vi "Lecture5exercise1.vi"() -> ()   [LabVIEW 2022 SP3]
uses:
  <vilib>/sound2/lvsound2.llb/Sampling Mode.ctl
  <vilib>/Analysis/2dsp.llb/Real FFT.vi
  <vilib>/sound2/lvsound2.llb/Sound Input Read (DBL).vi
  <vilib>/Analysis/NI_AALPro.lvlib
panel:
  out "Numeric":dbl
  out "Frequency Spectrum":cluster{dbl, dbl, dbl[]}(graph)
  out "Waveform Graph":waveform(dbl)(graph)
  in  "stop":bool
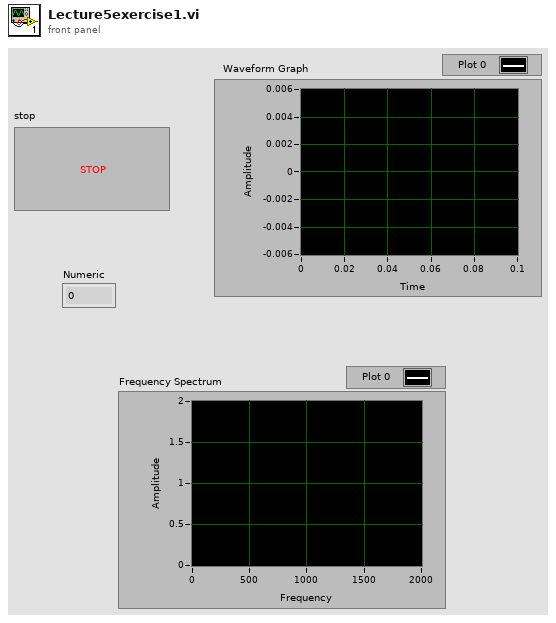
[diagram p1: front panel]
types:
  T1 = typedef "Sampling Mode.ctl" = i32
  T2 = typedef "Sound Input Task ID.ctl" = u32
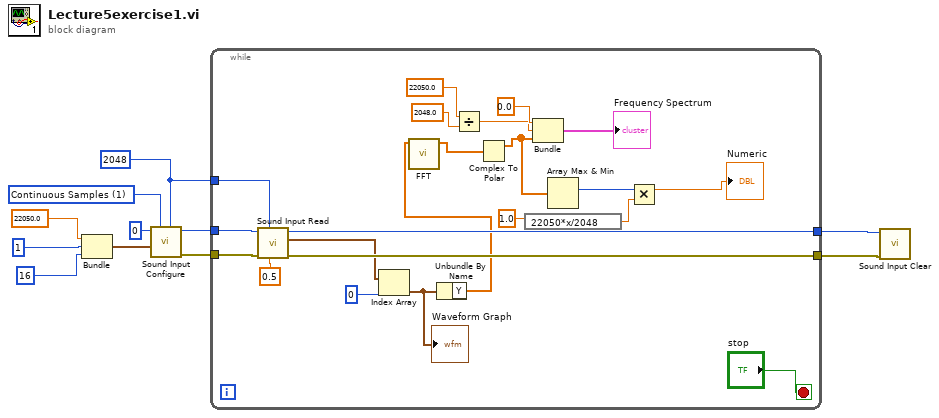
[diagram p0: block diagram]
diagram:
  w3 = 2048 ("number of samples/ch")
  w6 = T1 1 items=["Finite Samples", "Continuous Samples"] ("sample mode")
  n1 = Bundle(22050.0, 1, 16) -> (w8:cluster{dbl, i32, i32})  [unwired: 1 in]
  n2 = call <vilib>:"Sound Input Configure.vi"("number of samples/ch"=w3, "sample mode"=w6, "sound format"=w8, "device ID"=u32 0) -> ("error out"=w5:errorcluster, "task ID"=w4:T2)  [unwired: 6 in]
  n3 = while {
    tunnel: w5 -> [w29]
    tunnel: w4 -> [w28]
    tunnel: w3 -> [w27]
    tunnel: [w26] -> w2
    tunnel: [w25] -> w1
    stop <- "stop" stop-if-true
    n4 = call-poly <vilib>:"Sound Input Read.vi"("timeout (sec)"=0.5, "number of samples/ch"=w27, "error in (no error)"=w29, "task ID"=w28) -> ("error out"=w25:errorcluster, "data"=w24:waveform(dbl)[], "task ID out"=w26:T2)  [unwired: 5 in]
    n5 = Index Array(array=w24, index=0) -> (element=w30:waveform(dbl))
    "Waveform Graph" <- w30
    n6 = Unbundle By Name(w30) -> ("Y"=w22:dbl[])
    n7 = call-poly <vilib>:"FFT.vi"("X"=w22) -> ("FFT {X}"=w23:cdb[])  [unwired: 9 in, 1 out]
    n8 = Divide(x=22050.0, y=2048.0) -> (x/y=w20:dbl)
    n9 = Complex To Polar(r * e^(i*theta)=w23) -> (r=w16:dbl[])  [unwired: 1 out]
    n10 = expression code="22050*x/2048"(1.0) -> (w13:dbl)
    n11 = Bundle(0.0, w20, w16) -> (→"Frequency Spectrum":cluster{dbl, dbl, dbl[]})  [unwired: 1 in]
    n12 = Array Max & Min(array=w16) -> (max index (indices)=w15:i32)  [unwired: 3 out]
    n13 = Multiply(x=w15, y=w13) -> (x*y=→"Numeric":dbl)
  }
  n14 = call <vilib>:"Sound Input Clear.vi"("error in (no error)"=w1, "task ID"=w2) -> ()  [unwired: 9 in, 1 out]
